vi "remove_array_outliers 1-26-2018.vi"(7 "n standard devs to filter":dbl=0.0001 min=0.0001 max=10000.0 format="%0.2f", 10 "input array":dbl[](array[numeric])) -> (2 "filtered array out":dbl[](array[numeric]))   [LabVIEW 2014]
uses:
  <vilib>/Analysis/NI_AALBase.lvlib
panel:
  out "output mean":dbl format="%0.2f"
  out "input mean":dbl format="%0.2f"
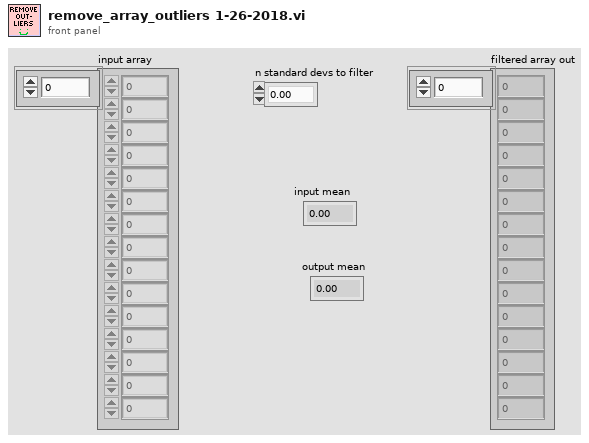
[diagram p1: front panel]
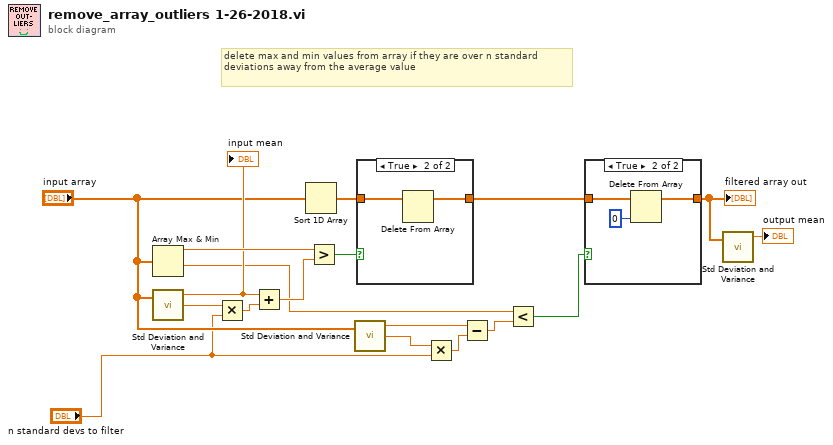
[diagram p0: block diagram]
diagram:
  # "delete max and min values from array if they are over n standard deviations away from the average value"
  n1 = Array Max & Min(array="input array") -> (max value=w18:dbl, min value=w9:dbl)  [unwired: 2 out]
  n2 = call <vilib>:"Std Deviation and Variance.vi"("X"="input array") -> ("mean"=w15:dbl, "standard deviation"=w17:dbl)  [unwired: 1 in, 1 out]
  "input mean" <- w15
  n3 = Multiply(x=w17, y="n standard devs to filter") -> (x*y=w16:dbl)
  n4 = Add(x=w15, y=w16) -> (x+y=w14:dbl)
  n5 = Sort 1D Array(array="input array") -> (sorted array=w12:dbl[])
  n6 = Greater?(x=w18, y=w14) -> (0:w13:bool)
  n7 = call <vilib>:"Std Deviation and Variance.vi"("X"="input array") -> ("mean"=w6:dbl, "standard deviation"=w11:dbl)  [unwired: 1 in, 1 out]
  n8 = case shown="True" w13 {
    tunnel: w12 -> [w19 w21]
    tunnel: [w19 w20] -> w4
    frame False {
    }
    frame True {
      n9 = Delete From Array(array=w21) -> (array with subset deleted=w20:dbl[])  [unwired: 2 in, 1 out]
    }
  }
  n10 = Multiply(x=w11, y="n standard devs to filter") -> (x*y=w10:dbl)
  n11 = Subtract(x=w6, y=w10) -> (x-y=w8:dbl)
  n12 = Less?(x=w9, y=w8) -> (x < y?=w5:bool)
  n13 = case shown="True" w5 {
    tunnel: w4 -> [w22 w25]
    tunnel: [w22 w24] -> w3
    frame False {
    }
    frame True {
      n14 = Delete From Array(array=w25, index=0) -> (array with subset deleted=w24:dbl[])  [unwired: 1 in, 1 out]
    }
  }
  "filtered array out" <- w3
  n15 = call <vilib>:"Std Deviation and Variance.vi"("X"=w3) -> ("mean"=→"output mean":dbl)  [unwired: 1 in, 2 out]
